vi "Echo Parameters.vi"   [LabVIEW 2015, in "Integration Tests.lvlib"]
uses:
  Integration Tests.lvlib
  LabVIEW Source/CLI Class/CLI.lvclass
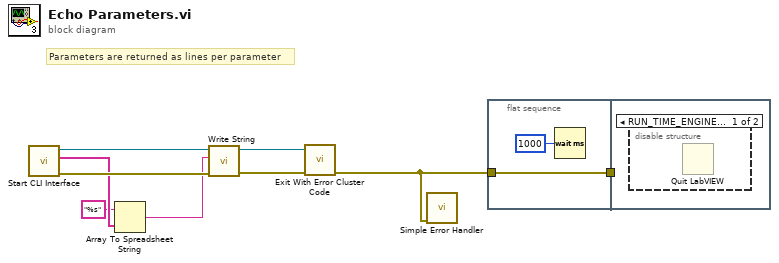
[diagram p0: block diagram]
diagram:
  # "Parameters are returned as lines per parameter"
  n1 = call "Start CLI Interface.vi"() -> ("error out"=w6:errorcluster, "Custom Parameters"=w5:string[], "CLI out"=w7:refnum<class "CLI.lvclass">)  [unwired: 8 in, 1 out]
  n2 = Array To Spreadsheet String(array=w5, 3:"%s" ("format string")) -> (spreadsheet string=w3:string)  [unwired: 1 in]
  n3 = call "Write String.vi"("error in (no error)"=w6, "Text to Write"=w3, "CLI in"=w7) -> ("error out"=w9:errorcluster, "CLI out"=w8:refnum<class "CLI.lvclass">)  [unwired: 7 in]
  n4 = call "Exit With Error Cluster Code.vi"("error in (no error)"=w9, "CLI in"=w8) -> ("error out"=w1:errorcluster)  [unwired: 9 in]
  n5 = call <vilib>:"Simple Error Handler.vi"("error in (no error)"=w1) -> ()  [unwired: 4 in, 5 out]
  n6 = flat-sequence {
    tunnel: w1 -> [w11]
    tunnel: [w11] -> w2
    tunnel: w2 -> [_]
    frame #0 {
      n7 = Wait (ms)(milliseconds to wait=u32 1000) -> ()  [unwired: 1 out]
    }
    frame #1 {
      n8 = disable-structure shown="RUN_TIME_ENGINE==True" {
        frame condition #0 {
          n9 = Quit LabVIEW() -> ()  [unwired: 1 in]
        }
        frame condition #1 (active) {
        }
      }
    }
  }
